vi "Convert user array to string table.vi"(3 "Expiration enabled":bool, 4 "User array":T1=[{"Active?"=TRUE, "User ID"="CTI", "Password"="CTI", "Name"="MIKE C", "Security level"=10, "Expired?"=FALSE, "Expire sec"=3100000000.0, "Locked?"=FALSE, "New?"=FALSE}] {"Expire sec" format="%.2f"}) -> (1 "Table":string[][](table)=[["CTI", "MIKE C", "10", "TRUE", "FALSE", "FALSE", "03/26/02 11:06:40 AM"]])   [LabVIEW 2012]
doc: "Converts the array of all users (access clusters) to a 2-D string table."
uses:
  User Access Type defs/User access cluster array.ctl
  User Access Type defs/User access cluster.ctl
  User Access Type defs/Security level U8.ctl
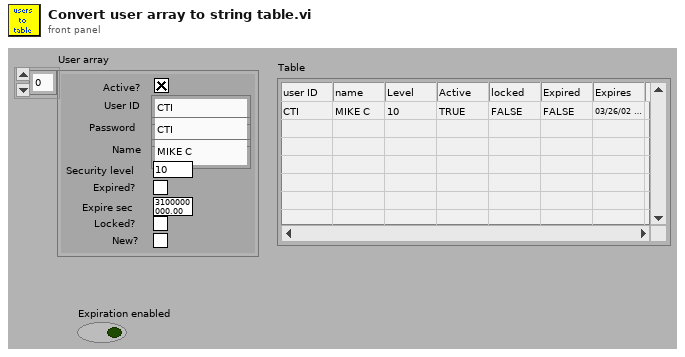
[diagram p1: front panel]
types:
  T1 = typedef "User access cluster array.ctl" = T2[]
  T2 = typedef "User access cluster.ctl" = cluster{"Active?":bool, "User ID":string, "Password":string, "Name":string, "Security level":T3, "Expired?":bool, "Expire sec":dbl, "Locked?":bool, "New?":bool}
  T3 = typedef "Security level U8.ctl" = u8
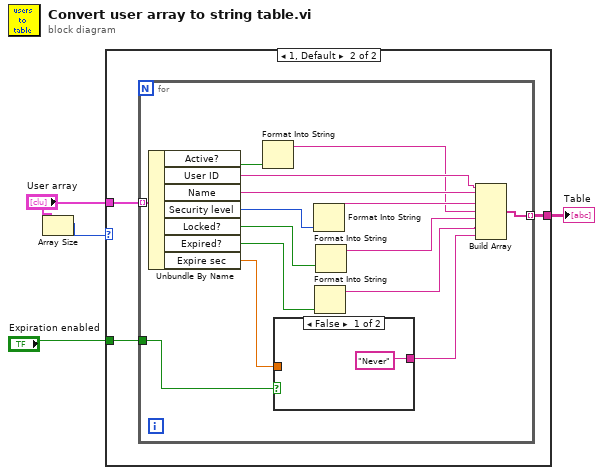
[diagram p0: block diagram]
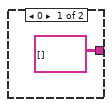
[diagram p2: hidden frame]
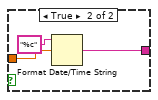
[diagram p3: hidden frame]
diagram:
  n1 = Array Size(array="User array") -> (size(s)=w3:i32)
  n2 = case shown="1, Default" w3 {
    tunnel: "User array" -> [_ w8]
    tunnel: [string[][] [] w7] -> w2
    tunnel: "Expiration enabled" -> [_ w6]
    frame 0 {
    }
    frame 1, Default {
      n3 = for {
        tunnel: w8 -> [w23] mode=indexing
        tunnel: [w21] -> w7 mode=indexing
        tunnel: w6 -> [w9]
        n4 = Unbundle By Name(w23) -> ("Active?"=w19:bool, "User ID"=w22:string, "Name"=w20:string, "Security level"=w18:T3, "Locked?"=w15:bool, "Expired?"=w13:bool, "Expire sec"=w11:dbl)
        n5 = Format Into String(w19) -> (resulting string=w16:string)  [unwired: 3 in, 1 out]
        n6 = case shown="False" w9 {
          tunnel: w11 -> [_ w27]
          tunnel: ["Never" ("date/time string") w25] -> w10
          frame False {
          }
          frame True {
            n7 = Format Date/Time String(time format string (%c)="%c", seconds (now)=w27) -> (date/time string=w25:string)  [unwired: 1 out]
          }
        }
        n8 = Format Into String(w18) -> (resulting string=w17:string)  [unwired: 3 in, 1 out]
        n9 = Format Into String(w13) -> (resulting string=w12:string)  [unwired: 3 in, 1 out]
        n10 = Format Into String(w15) -> (resulting string=w14:string)  [unwired: 3 in, 1 out]
        n11 = Build Array(w22, w20, w17, w16, w14, w12, w10) -> (w21:string[])
      }
    }
  }
  "Table" <- w2
